vi "Get SMO HELP getAll.vi"(8 "error in (no error)":errorcluster, 11 "Inst.RP100 in":refnum<class "Inst.RP100.lvclass">) -> (0 "error out":errorcluster, 1 "response info table":string[][](array[string])=[["name", "description"], ["*", "*"]], 2 "response cluster":variant, 3 "Inst.RP100 out":refnum<class "Inst.RP100.lvclass">)   [LabVIEW 2019, in "Inst.RP100.lvclass"]
uses:
  Inst.RP100.lvclass
  Typedefs/Inst.RP100.getAll--Cluster.ctl
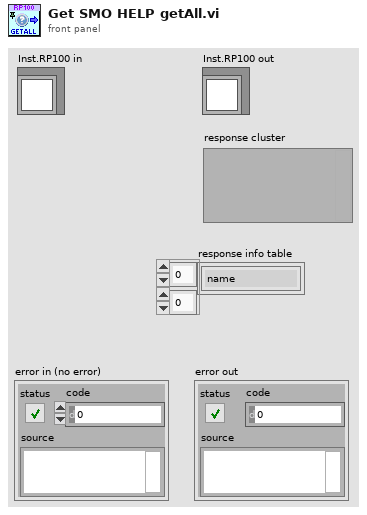
[diagram p1: front panel]
types:
  T1 = typedef "Inst.RP100.lvclass/Inst.RP100.getAll--Cluster.ctl" = cluster{"OutputStateCh1":string, "OutputStateCh2":string, "LevelCh1":dbl, "LevelCh2":dbl, "SlewCh1":dbl, "SlewCh2":dbl, "MeasuredVCh1":dbl, "MeasuredVCh2":dbl, "MeasuredICh1":dbl, "MeasuredICh2":dbl}
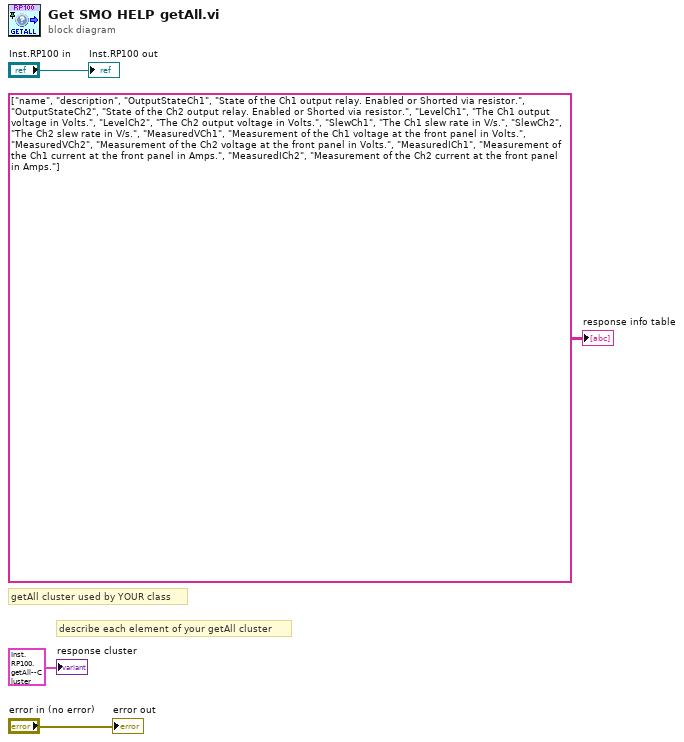
[diagram p0: block diagram]
diagram:
  # "describe each element of your getAll cluster"
  # "getAll cluster used by YOUR class"
  "Inst.RP100 out" <- "Inst.RP100 in"
  "response info table" <- string[][] [["name", "description"], ["OutputStateCh1", "State of the Ch1 output relay. Enabled or Shorted via resistor."], ["OutputStateCh2", "State of the Ch2 output relay. Enabled or Shorted via resistor."], ["LevelCh1", "The Ch1 output voltage in Volts."], ["LevelCh2", "The Ch2 output voltage in Volts."], ["SlewCh1", "The Ch1 slew rate in V/s."], ["SlewCh2", "The Ch2 slew rate in V/s."], ["MeasuredVCh1", "Measurement of the Ch1 voltage at the front panel in Volts."], ["MeasuredVCh2", "Measurement of the Ch2 voltage at the front panel in Volts."], ["MeasuredICh1", "Measurement of the Ch1 current at the front panel in Amps."], ["MeasuredICh2", "Measurement of the Ch2 current at the front panel in Amps."]] ("response/request info table: description of request or reponse cluster")
  "error out" <- "error in (no error)"
  "response cluster" <- T1 {"OutputStateCh1"="", "OutputStateCh2"="", "LevelCh1"=0.0, "LevelCh2"=0.0, "SlewCh1"=0.0, "SlewCh2"=0.0, "MeasuredVCh1"=0.0, "MeasuredVCh2"=0.0, "MeasuredICh1"=0.0, "MeasuredICh2"=0.0} ("getAll")
